vi "Global 1.vi"() -> ()   [LabVIEW 2020]
panel:
  in  "GlobalVariable":dbl
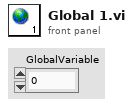
[diagram p1: front panel]
diagram:
